vi "Write ExperimentStats.vi"(8 "error in (no error)":errorcluster, 10 "ExperimentStats":T1, 11 "TrialBasedExperiment in":refnum<class "TrialBasedExperiment.lvclass">) -> (0 "error out":errorcluster, 3 "TrialBasedExperiment out":refnum<class "TrialBasedExperiment.lvclass">)   [LabVIEW 2014, in "AcquisitionCoreObjects.lvlib" / "TrialBasedExperiment.lvclass"]
uses:
  TrialBasedExperiment.lvclass
  TrialBasedExperiment.lvclass/TrialBasedExperiment.ctl
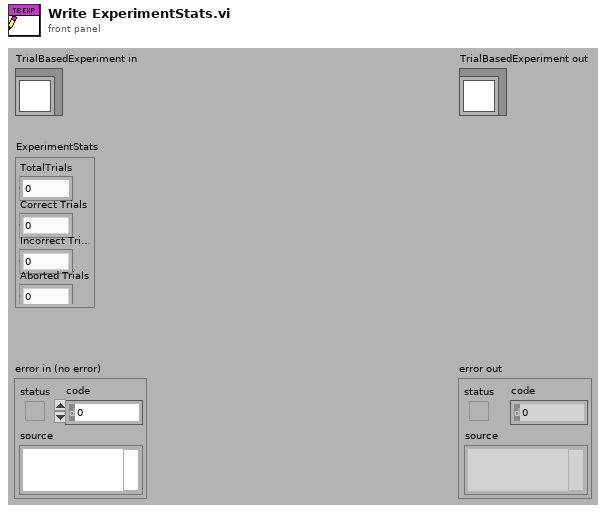
[diagram p1: front panel]
types:
  T1 = cluster{"TotalTrials":u32, "Correct Trials":u32, "Incorrect Trials":u32, "Aborted Trials":u32}
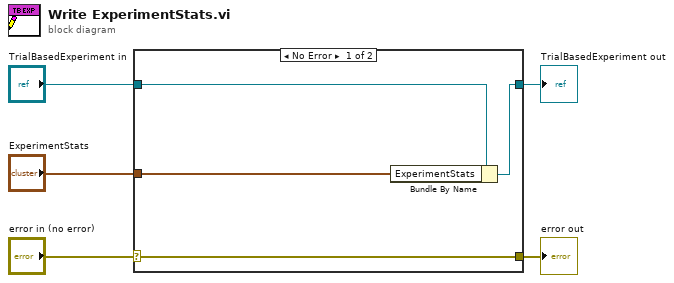
[diagram p0: block diagram]
diagram:
  n1 = case shown="No Error" "error in (no error)" {
    selector: "error in (no error)" -> [w9 w10]
    tunnel: [w9 w10] -> w4
    tunnel: [w7 w11] -> w2
    tunnel: "TrialBasedExperiment in" -> [w8 w11]
    tunnel: "ExperimentStats" -> [w6 _]
    frame No Error {
      n2 = Bundle By Name(cluster=w8, "ExperimentStats"=w6) -> (w7:refnum<class "TrialBasedExperiment.lvclass">)
    }
    frame Error {
    }
  }
  "error out" <- w4
  "TrialBasedExperiment out" <- w2
